vi "Format Message For Write.vi"(7 "generate error if invalid (T)":bool=TRUE, 8 "error in":errorcluster, 9 "meta data":T1[](array[typedef]), 10 "data":string, 11 "message name":string) -> (0 "error out":errorcluster, 1 "valid?":bool, 3 "message":string)   [LabVIEW 2013, in "NI STM.lvlib"]
uses:
  NI STM.lvlib
  MetaDataElement.ctl
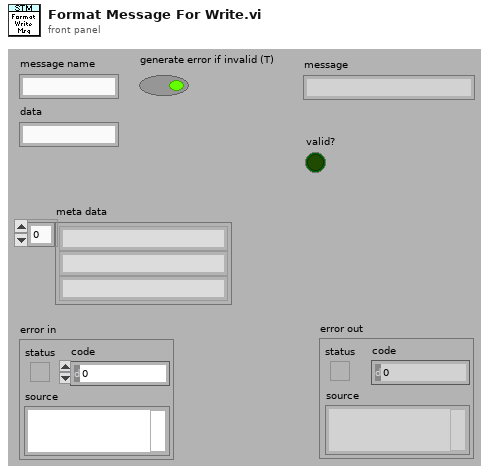
[diagram p1: front panel]
types:
  T1 = typedef "NI STM.lvlib/MetaDataElement.ctl" = string
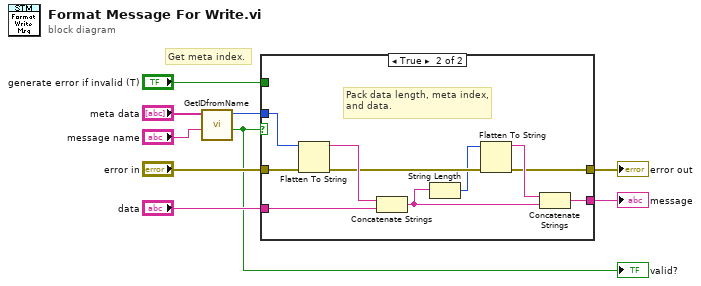
[diagram p0: block diagram]
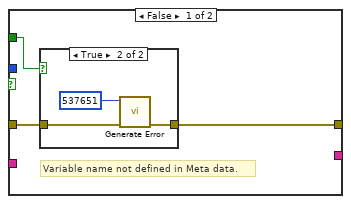
[diagram p2: hidden frame]
diagram:
  # "Get meta index."
  n1 = call "GetIDfromName.vi"("name"="message name", "meta data"="meta data") -> ("found?"=w1:bool, "meta ID"=w7:u16)  [unwired: 8 out]
  "valid?" <- w1
  n2 = case shown="True" w1 {
    tunnel: w7 -> [_ w25]
    tunnel: "data" -> [_ w23]
    tunnel: "error in" -> [w12 w26]
    tunnel: [_ w18] -> w4
    tunnel: [w11 w17] -> w3
    tunnel: "generate error if invalid (T)" -> [w10 _]
    frame False {
      # "Variable name not defined in Meta data."
      n3 = case shown="True" w10 {
        tunnel: w12 -> [w13 w16]
        tunnel: [w13 w14] -> w11
        frame False {
        }
        frame True {
          n4 = call "Generate Error.vi"("error in"=w16, "code"=537651) -> ("error out"=w14:errorcluster)  [unwired: 9 in]
        }
      }
    }
    frame True {
      # "Pack data length, meta index, and data."
      n5 = Flatten To String(anything=w25, error in (no error)=w26) -> (data string=w24:string, error out=w22:errorcluster)  [unwired: 3 out]
      n6 = Concatenate Strings(w24, w23) -> (w19:string)
      n7 = String Length(string=w19) -> (length=w21:i32)
      n8 = Flatten To String(anything=w21, error in (no error)=w22) -> (data string=w20:string, error out=w17:errorcluster)  [unwired: 3 out]
      n9 = Concatenate Strings(w20, w19) -> (w18:string)
    }
  }
  "error out" <- w3
  "message" <- w4
